vi "Compile IO.vi"(8 "error in (no error)":errorcluster, 9 "IO Control":T1[](array[typedef]) {"Signals"."Response"."Byte Order" items=["Little Endian", "Big Endian"]; "Signals"."Response"."Data Type" items=["Signed", "Unsigned", "IEEE Float"]; "Signals"."Cmd"."Byte Order" items=["Little Endian", "Big Endian"]; "Signals"."Cmd"."Data Type" items=["Signed", "Unsigned", "IEEE Float"]}, 10 "IO Refs":T4[](array[typedef]) {"Signals"."Cmd Refs" format="%.0x"; "Signals"."Resp Refs" format="%.0x"}, 11 "Item Ref in":T6 format="%.0x") -> (0 "error out":errorcluster, 1 "Cmd Refs":cluster{"Refs":T8[], "Values":dbl[]} {"Refs"."Data Reference" format="%.0x"}, 2 "Cmd Lookup Table":variant, 3 "Item Ref out":T6=18446744073709551615 format="%.0x", 4 "Resp Lookup Table":variant, 6 "Resp Refs":T7[](array[typedef]) format="%.0x")   [LabVIEW 2015, in "Diagnostics Addon System Explorer.lvlib"]
uses:
  Diagnostics Addon System Explorer.lvlib
  <vilib>/NI Veristand/Custom Device API/Custom Device Item Ref.ctl
  <vilib>/NI Veristand/Custom Device API/Block Data Reference.ctl
  <vilib>/NI Veristand/Custom Device API/Data Reference.ctl
  Types/IO VS References.ctl
  Shared/Types/CmdResp Refs.ctl
  Shared/Types/IO Control Parameters.ctl
  Shared/Types/Command Response Signals.ctl
  Shared/Types/Signal Parameters.ctl
  <vilib>/NI Veristand/Custom Device API/Data Access Type.ctl
  Shared/Types/Datatable Lookup Positions.ctl
  Shared/Diagnostics Addon Shared.lvlib
  <vilib>/NI Veristand/Custom Device API/Custom Device API.lvlib
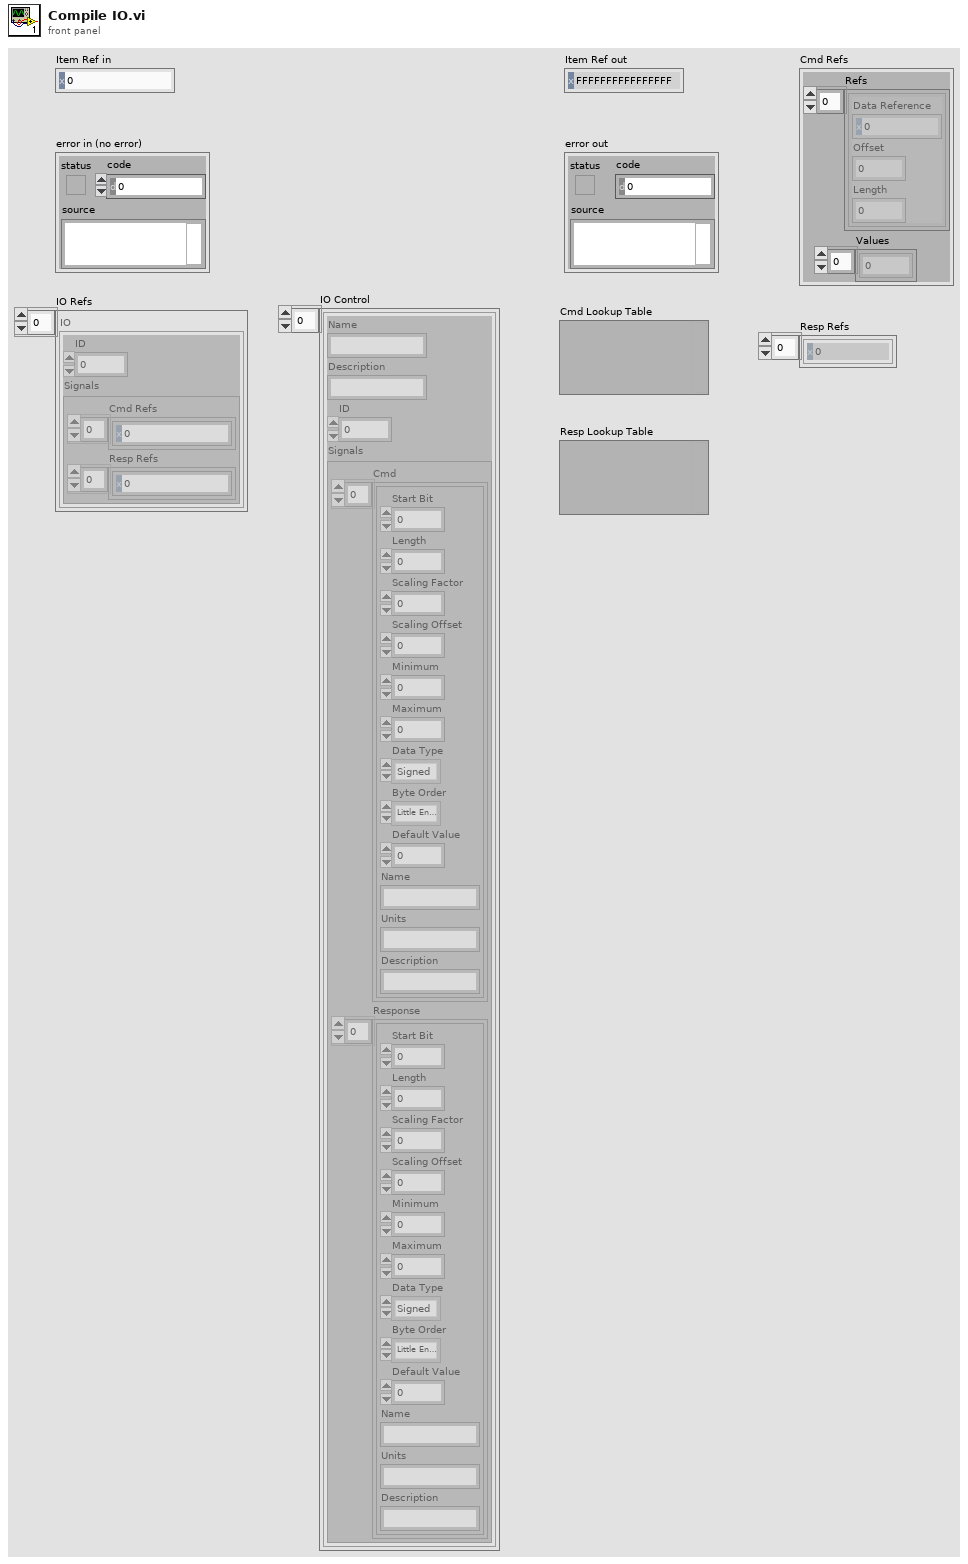
[diagram p1: front panel]
types:
  T1 = typedef "Diagnostics Addon Shared.lvlib/IO Control Parameters.ctl" = cluster{"Name":string, "Description":string, "ID":u16, "Signals":T2}
  T2 = typedef "Diagnostics Addon Shared.lvlib/Command Response Signals.ctl" = cluster{"Cmd":T3[], "Response":T3[]}
  T3 = typedef "Diagnostics Addon Shared.lvlib/Signal Parameters.ctl" = cluster{"Start Bit":u8, "Length":u8, "Scaling Factor":dbl, "Scaling Offset":dbl, "Minimum":dbl, "Maximum":dbl, "Data Type":u32, "Byte Order":u32, "Default Value":dbl, "Name":string, "Units":string, "Description":string}
  T4 = typedef "Diagnostics Addon System Explorer.lvlib/IO VS References.ctl" = cluster{"ID":u32, "Signals":T5}
  T5 = typedef "Diagnostics Addon Shared.lvlib/CmdResp Refs.ctl" = cluster{"Cmd Refs":T6[], "Resp Refs":T6[]}
  T6 = typedef "Custom Device API.lvlib/Custom Device Item Ref.ctl" = u64
  T7 = typedef "Custom Device API.lvlib/Data Reference.ctl" = i32
  T8 = typedef "Custom Device API.lvlib/Block Data Reference.ctl" = cluster{"Data Reference":T7, "Offset":u64, "Length":u64}
  T9 = typedef "Custom Device API.lvlib/Data Access Type.ctl" = enum16{"Read", "Write"}
  T10 = typedef "Diagnostics Addon Shared.lvlib/Datatable Lookup Positions.ctl" = cluster{"Offset":i32, "Length":i32, "ByteLength":u16}
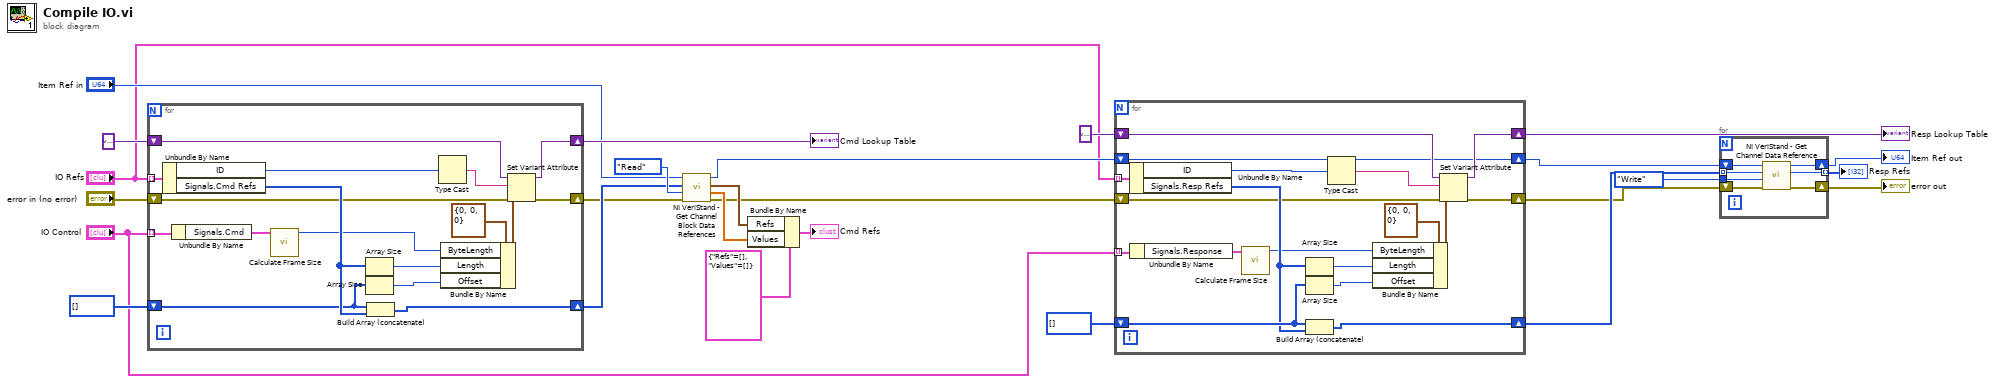
[diagram p0: block diagram]
diagram:
  n1 = for {
    tunnel: "IO Refs" -> [w35] mode=indexing
    shift-right: [w36] -> w24
    shift-left: variant -> [w40]
    shift-right: [w38] -> w16
    shift-left: "error in (no error)" -> [w31]
    shift-right: [w34] -> w21
    shift-left: T6[] [] -> [w32]
    tunnel: "IO Control" -> [w30] mode=indexing
    n2 = Unbundle By Name(w35) -> ("ID"=w27:u32, "Signals.Cmd Refs"=w33:T6[])
    n3 = Unbundle By Name(w30) -> ("Signals.Cmd"=w29:T3[])
    n4 = call "Calculate Frame Size.vi"("Parameters"=w29) -> ("Bytes"=w28:u16)  [unwired: 10 in]
    n5 = Array Size(array=w33) -> (size(s)=w43:i32)
    n6 = Array Size(array=w32) -> (size(s)=w39:i32)
    n7 = Build Array (concatenate)(w32, w33) -> (w34:T6[])
    n8 = Type Cast(x=w27) -> (*(type *) &x=w37:string)  [unwired: 1 in]
    n9 = Bundle By Name(cluster=T10 {"Offset"=0, "Length"=0, "ByteLength"=0}, "ByteLength"=w28, "Length"=w43, "Offset"=w39) -> (w41:T10)
    n10 = Set Variant Attribute(Variant=w40, name=w37, value=w41, error in=w31) -> (Variant out=w36:variant, error out=w38:errorcluster)  [unwired: 1 out]
  }
  "Cmd Lookup Table" <- w24
  n11 = call <vilib>:"NI VeriStand - Get Channel Block Data References.vi"("error in (no error)"=w16, "Access"=Data_Access_Type."Read", "Channel Refs"=w21, "Device Ref in"="Item Ref in") -> ("error out"=w5:errorcluster, "Values Array"=w17:dbl[], "Block Data Refs"=w18:T8[], "Device Ref out"=w4:T6)  [unwired: 4 in]
  n12 = Bundle By Name(cluster=cluster{"Refs":T8[], "Values":dbl[]} {"Refs"=[], "Values"=[]} ("Pairs"), "Refs"=w18, "Values"=w17) -> (→"Cmd Refs":cluster{"Refs":T8[], "Values":dbl[]})
  n13 = for {
    tunnel: "IO Refs" -> [w51] mode=indexing
    shift-right: [w60] -> w9
    shift-left: T6[] [] ("Signal Refs") -> [w61]
    shift-right: [w52] -> w13
    shift-left: variant -> [w56]
    shift-right: [w54] -> w8
    shift-left: w5 -> [w49]
    shift-right: [w48] -> w10
    shift-left: w4 -> [w48]
    tunnel: "IO Control" -> [w47] mode=indexing
    n14 = Unbundle By Name(w51) -> ("ID"=w44:u32, "Signals.Resp Refs"=w50:T6[])
    n15 = Unbundle By Name(w47) -> ("Signals.Response"=w46:T3[])
    n16 = call "Calculate Frame Size.vi"("Parameters"=w46) -> ("Bytes"=w45:u16)  [unwired: 10 in]
    n17 = Array Size(array=w50) -> (size(s)=w59:i32)
    n18 = Array Size(array=w61) -> (size(s)=w55:i32)
    n19 = Build Array (concatenate)(w61, w50) -> (w60:T6[])
    n20 = Type Cast(x=w44) -> (*(type *) &x=w53:string)  [unwired: 1 in]
    n21 = Bundle By Name(cluster=T10 {"Offset"=0, "Length"=0, "ByteLength"=0}, "ByteLength"=w45, "Length"=w59, "Offset"=w55) -> (w57:T10)
    n22 = Set Variant Attribute(Variant=w56, name=w53, value=w57, error in=w49) -> (Variant out=w52:variant, error out=w54:errorcluster)  [unwired: 1 out]
  }
  "Resp Lookup Table" <- w13
  n23 = for {
    tunnel: w9 -> [w64] mode=indexing
    tunnel: Data_Access_Type."Write" ("Access") -> [w63]
    shift-right: [w66] -> w1
    shift-left: w8 -> [w67]
    shift-right: [w68] -> w2
    shift-left: w10 -> [w65]
    tunnel: [w62] -> w7 mode=indexing
    n24 = call <vilib>:"NI VeriStand - Get Channel Data Reference.vi"("error in (no error)"=w67, "Access"=w63, "Channel Ref in"=w64, "Device Ref in"=w65) -> ("error out"=w66:errorcluster, "Channel Data Reference"=w62:T7, "Device Ref out"=w68:T6)  [unwired: 5 in]
  }
  "error out" <- w1
  "Item Ref out" <- w2
  "Resp Refs" <- w7
